vi "Swerve Drive.vi"(0 "X":dbl(slide) scale=-1.0..1.0, 1 "Rot. Point Y":dbl, 3 "Rot. Point X":dbl, 4 "Back Left":bool, 6 "Back Right":bool, 7 "Y":dbl(slide) scale=1.0..-1.0, 8 "Front Left":bool, 10 "Front Right":bool, 11 "Z":dbl(knob) scale=1.0..-1.0, 12 "Auto Controls":bool, 13 "Robot-Centric":bool) -> (15 "Debug is on":bool)   [LabVIEW 2016]
uses:
  Swerve Testing 2017/Added Files/Apple Gyro/Apple Pi Gyro Library.lvlib
panel:
  in  "Deadband":dbl=0.04 format="%#_13g"
  in  "Robot Length":dbl=21.5
  in  "Robot Width":dbl=29.5
  # "SWERVE DRIVE\nVersion 3.2\n\nCory Lynch\nChris Garuti\nApple Pi Robotics\nTeam 2067"
  # "Debug"
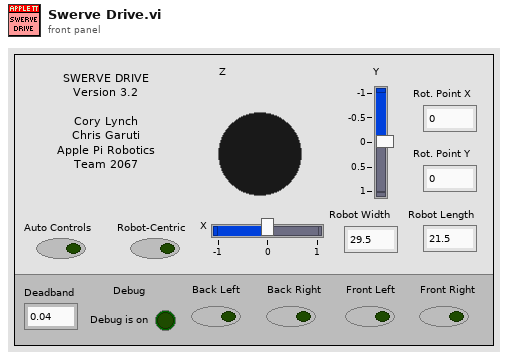
[diagram p1: front panel]
types:
  T1 = enum16{"Back Left", "Back Right", "Front Left", "Front Right"}
  T2 = typedef "WPI_MotorControlDeviceRef.ctl" = cluster{"DeviceStatus":errorcluster, "Type":T3, "PWM":cluster{"PWM Channel":T4, "DeadBand":T5}, "CAN":cluster{"Device Number":u8, "SetOutput VI Ref":variant, "GetOutput VI Ref":variant, "Enable VI Ref":variant, "Disable VI Ref":variant, "Data":variant}, "Invert":bool}
  T3 = typedef "WPI_MotorControlType.ctl" = enum16{"PWM", "CAN"}
  T4 = typedef "FPGA_DIOPWMChannel.ctl" = enum8{"PWM 0", "PWM 1", "PWM 2", "PWM 3", "PWM 4", "PWM 5", "PWM 6", "PWM 7", "PWM 8", "PWM 9", "PWM MXP 0", "PWM MXP 1", "PWM MXP 2", "PWM MXP 3", "PWM MXP 4", "PWM MXP 5", "PWM MXP 6", "PWM MXP 7", "PWM MXP 8", "PWM MXP 9", "Invalid"}
  T5 = typedef "WPI_PWMDeadband.ctl" = cluster{"Name":string, "maxPositivePwm":i32, "minPositivePwm":i32, "centerPwm":i32, "maxNegativePwm":i32, "minNegativePwm":i32, "angularRange":u16}
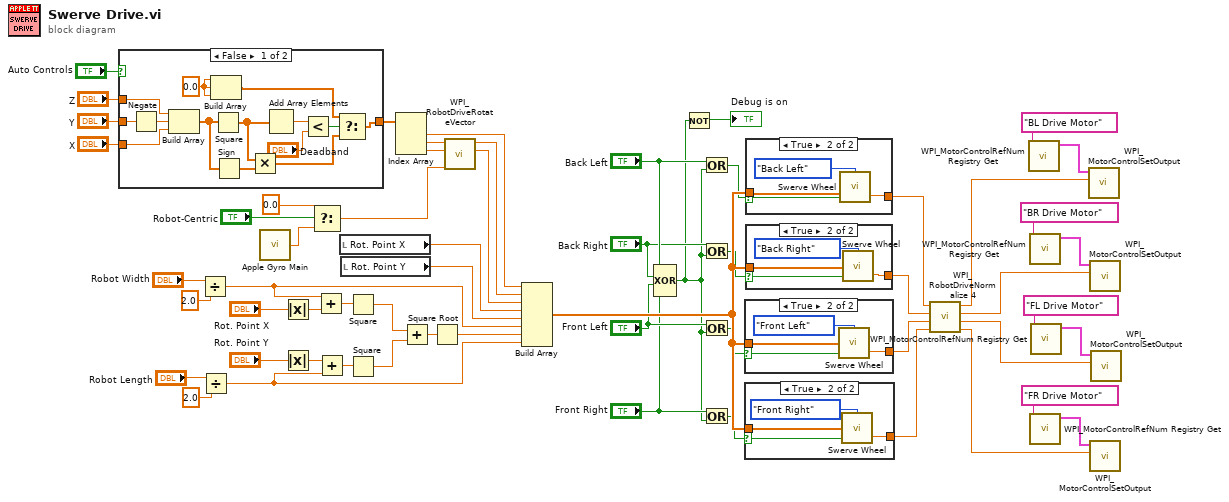
[diagram p0: block diagram]
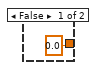
[diagram p2: hidden frame]
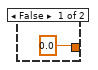
[diagram p3: hidden frame]
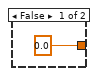
[diagram p4: hidden frame]
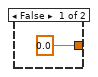
[diagram p5: hidden frame]
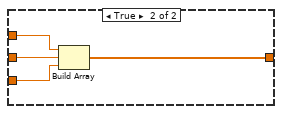
[diagram p6: hidden frame]
diagram:
  n1 = case shown="False" "Auto Controls" {
    tunnel: "Y" -> [w70 w76]
    tunnel: "X" -> [w64 w77]
    tunnel: "Z" -> [w60 w74]
    tunnel: [w61 w75] -> w20
    frame False {
      w68 = 0.0 ("element")
      n2 = Negate(x=w70) -> (-x=w63:dbl)
      n3 = Build Array(w60, w63, w64) -> (w67:dbl[])
      n4 = Build Array(w68, w68, w68) -> (w69:dbl[])
      n5 = Square(x=w67) -> (x^2=w65:dbl[])
      n6 = Sign(1:w67) -> (0:w66:dbl[])
      n7 = Multiply(x=w65, y=w66) -> (x*y=w62:dbl[])
      n8 = Add Array Elements(numeric array=w65) -> (sum=w73:dbl)
      n9 = Less?(x=w73, y="Deadband") -> (x < y?=w71:bool)
      n10 = Select(t=w69, s=w71, f=w62) -> (s? t:f=w61:dbl[])
    }
    frame True {
      n11 = Build Array(w74, w76, w77) -> (w75:dbl[])
    }
  }
  n12 = Divide(x="Robot Width", y=2.0) -> (x/y=w24:dbl)
  n13 = Divide(x="Robot Length", y=2.0) -> (x/y=w22:dbl)
  n14 = call "Apple Gyro Main.vi"() -> ("Gyro Yaw Out"=w11:dbl)  [unwired: 4 in]
  n15 = Absolute Value(x="Rot. Point X") -> (abs(x)=w42:dbl)
  n16 = Absolute Value(x="Rot. Point Y") -> (abs(x)=w40:dbl)
  n17 = Select(t=0.0, s="Robot-Centric", f=w11) -> (s? t:f=w15:dbl)
  n18 = Add(x=w24, y=w42) -> (x+y=w41:dbl)
  n19 = Add(x=w40, y=w22) -> (x+y=w39:dbl)
  n20 = local read "Rot. Point X"() -> (w26:dbl)
  n21 = local read "Rot. Point Y"() -> (w25:dbl)
  n22 = Square(x=w41) -> (x^2=w37:dbl)
  n23 = Square(x=w39) -> (x^2=w38:dbl)
  n24 = Index Array(array=w20) -> (element #1=w14:dbl, element #2=w21:dbl, element #3=w29:dbl)  [unwired: 3 in]
  n25 = Add(x=w37, y=w38) -> (x+y=w36:dbl)
  n26 = Square Root(x=w36) -> (sqrt(x)=w23:dbl)
  n27 = call <vilib>:"WPI_RobotDriveRotateVector.vi"("Angle"=w15, "X"=w29, "Y"=w21) -> ("X'"=w18:dbl, "Y'"=w13:dbl)  [unwired: 7 out]
  n28 = Build Array(w14, w13, w18, w26, w25, w24, w23, w22) -> (w19:dbl[])
  n29 = Compound Arithmetic op=XOR("Back Left", "Back Right", "Front Left", "Front Right") -> (w2:bool)
  n30 = Not(x=w2) -> (.not. x?=→"Debug is on":bool)
  n31 = Or(x="Back Left", y=w2) -> (x .or. y?=w10:bool)
  n32 = Or(x="Back Right", y=w2) -> (x .or. y?=w9:bool)
  n33 = Or(x="Front Left", y=w2) -> (x .or. y?=w8:bool)
  n34 = Or(x="Front Right", y=w2) -> (x .or. y?=w7:bool)
  n35 = case shown="True" w8 {
    selector: w8 -> [_ w79]
    tunnel: [0.0 ("Speed") w81] -> w57
    tunnel: w19 -> [_ w80]
    frame False {
    }
    frame True {
      n36 = call "Swerve Wheel.vi"("Wheel"=T1."Front Left", "Debug?"=w79, "Inputs"=w80) -> ("Speed"=w81:dbl)  [unwired: 2 in]
    }
  }
  n37 = case shown="True" w7 {
    selector: w7 -> [_ w84]
    tunnel: [0.0 ("Speed") w86] -> w56
    tunnel: w19 -> [_ w85]
    frame False {
    }
    frame True {
      n38 = call "Swerve Wheel.vi"("Wheel"=T1."Front Right", "Debug?"=w84, "Inputs"=w85) -> ("Speed"=w86:dbl)  [unwired: 2 in]
    }
  }
  n39 = case shown="True" w10 {
    selector: w10 -> [_ w89]
    tunnel: [0.0 ("Speed") w92] -> w59
    tunnel: w19 -> [_ w90]
    frame False {
    }
    frame True {
      n40 = call "Swerve Wheel.vi"("Wheel"=T1."Back Left", "Debug?"=w89, "Inputs"=w90) -> ("Speed"=w92:dbl)  [unwired: 2 in]
    }
  }
  n41 = case shown="True" w9 {
    selector: w9 -> [_ w94]
    tunnel: [0.0 ("Speed") w96] -> w58
    tunnel: w19 -> [_ w95]
    frame False {
    }
    frame True {
      n42 = call "Swerve Wheel.vi"("Wheel"=T1."Back Right", "Debug?"=w94, "Inputs"=w95) -> ("Speed"=w96:dbl)  [unwired: 2 in]
    }
  }
  n43 = call <vilib>:"WPI_RobotDriveNormalize 4.vi"("D"=w56, "C"=w57, "B"=w58, "A"=w59) -> ("D'"=w44:dbl, "C'"=w45:dbl, "B'"=w46:dbl, "A'"=w47:dbl)
  n44 = call <vilib>:"WPI_MotorControlRefNum Registry Get.vi"("refnum name"="BL Drive Motor") -> ("MotorControlDevRef"=w55:T2)  [unwired: 9 in, 1 out]
  n45 = call <vilib>:"WPI_MotorControlRefNum Registry Get.vi"("refnum name"="BR Drive Motor") -> ("MotorControlDevRef"=w52:T2)  [unwired: 9 in, 1 out]
  n46 = call <vilib>:"WPI_MotorControlRefNum Registry Get.vi"("refnum name"="FR Drive Motor") -> ("MotorControlDevRef"=w48:T2)  [unwired: 9 in, 1 out]
  n47 = call <vilib>:"WPI_MotorControlRefNum Registry Get.vi"("refnum name"="FL Drive Motor") -> ("MotorControlDevRef"=w51:T2)  [unwired: 9 in, 1 out]
  n48 = call <vilib>:"WPI_MotorControlSetOutput.vi"("Output"=w47, "MotorControlDevRef"=w55) -> ()  [unwired: 7 in, 3 out]
  n49 = call <vilib>:"WPI_MotorControlSetOutput.vi"("Output"=w46, "MotorControlDevRef"=w52) -> ()  [unwired: 7 in, 3 out]
  n50 = call <vilib>:"WPI_MotorControlSetOutput.vi"("Output"=w44, "MotorControlDevRef"=w48) -> ()  [unwired: 7 in, 3 out]
  n51 = call <vilib>:"WPI_MotorControlSetOutput.vi"("Output"=w45, "MotorControlDevRef"=w51) -> ()  [unwired: 7 in, 3 out]
